vi "ASCII String To Data.vi"   [LabVIEW 2016, in "CVT.lvlib" / "Current Value Table.lvlib"]
doc: "This VI converts data stored on disk as an ascii string into the correct data type. This VI must perform the opposite operation to the Data To ASCII String function."
uses:
  <vilib>/NI/Current Value Table/Current Value Table.lvlib
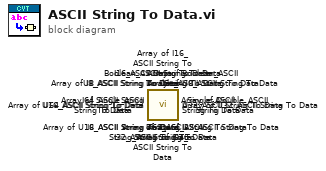
[diagram p0: block diagram]
diagram:
  n1 = call <vilib>:"Array of String_ASCII String To Data.vi"() -> ()  [unwired: 10 in, 2 out]
  n2 = call <vilib>:"Array of Boolean_ASCII String To Data.vi"() -> ()  [unwired: 10 in, 2 out]
  n3 = call <vilib>:"Array of Single_ASCII String To Data.vi"() -> ()  [unwired: 10 in, 2 out]
  n4 = call <vilib>:"Array of Double_ASCII String To Data.vi"() -> ()  [unwired: 10 in, 2 out]
  n5 = call <vilib>:"Array of I8_ASCII String To Data.vi"() -> ()  [unwired: 10 in, 2 out]
  n6 = call <vilib>:"Array of I16_ASCII String To Data.vi"() -> ()  [unwired: 10 in, 2 out]
  n7 = call <vilib>:"Array of I32_ASCII String To Data.vi"() -> ()  [unwired: 10 in, 2 out]
  n8 = call <vilib>:"Array of I64_ASCII String To Data.vi"() -> ()  [unwired: 10 in, 2 out]
  n9 = call <vilib>:"Array of U64_ASCII String To Data.vi"() -> ()  [unwired: 10 in, 2 out]
  n10 = call <vilib>:"Array of U32_ASCII String To Data.vi"() -> ()  [unwired: 10 in, 2 out]
  n11 = call <vilib>:"Array of U16_ASCII String To Data.vi"() -> ()  [unwired: 10 in, 2 out]
  n12 = call <vilib>:"Array of U8_ASCII String To Data.vi"() -> ()  [unwired: 10 in, 2 out]
  n13 = call <vilib>:"Boolean_ASCII String To Data.vi"() -> ()  [unwired: 10 in, 2 out]
  n14 = call <vilib>:"String_ASCII String To Data.vi"() -> ()  [unwired: 10 in, 2 out]
  n15 = call <vilib>:"U8_ASCII String To Data.vi"() -> ()  [unwired: 10 in, 2 out]
  n16 = call <vilib>:"U16_ASCII String To Data.vi"() -> ()  [unwired: 10 in, 2 out]
  n17 = call <vilib>:"U32_ASCII String To Data.vi"() -> ()  [unwired: 10 in, 2 out]
  n18 = call <vilib>:"U64_ASCII String To Data.vi"() -> ()  [unwired: 10 in, 2 out]
  n19 = call <vilib>:"I8_ASCII String To Data.vi"() -> ()  [unwired: 10 in, 2 out]
  n20 = call <vilib>:"I16_ASCII String To Data.vi"() -> ()  [unwired: 10 in, 2 out]
  n21 = call <vilib>:"I32_ASCII String To Data.vi"() -> ()  [unwired: 10 in, 2 out]
  n22 = call <vilib>:"I64_ASCII String To Data.vi"() -> ()  [unwired: 10 in, 2 out]
  n23 = call <vilib>:"Single_ASCII String To Data.vi"() -> ()  [unwired: 10 in, 2 out]
  n24 = call <vilib>:"Double_ASCII String To Data.vi"() -> ()  [unwired: 10 in, 2 out]
